vi "CRC.vi"(7 "Byte_order":enum16{"Windows", "DSP"}(ring), 10 "String in":string) -> (1 "CRC16":string, 2 "CRC16":u16 format="%04x", 4 "calculated from #":i32)   [LabVIEW 2017, in "ZBOX_IS.lvlib"]
uses:
  ZBOX_IS.lvlib
panel:
  out "Data in 2":u16[](array[numeric]) format="%02x"
  out "Data in":u8[](array[numeric]) format="%02x"
  out "Data in":u8[](array[numeric]) format="%02x"
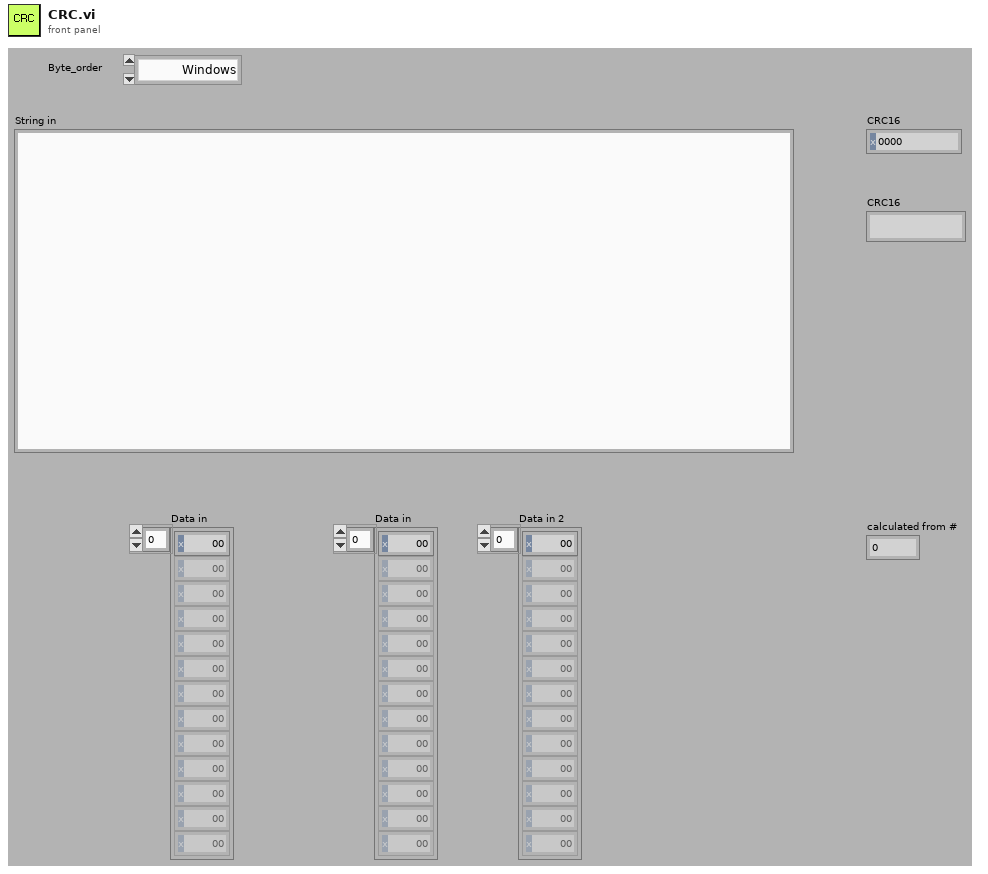
[diagram p1: front panel]
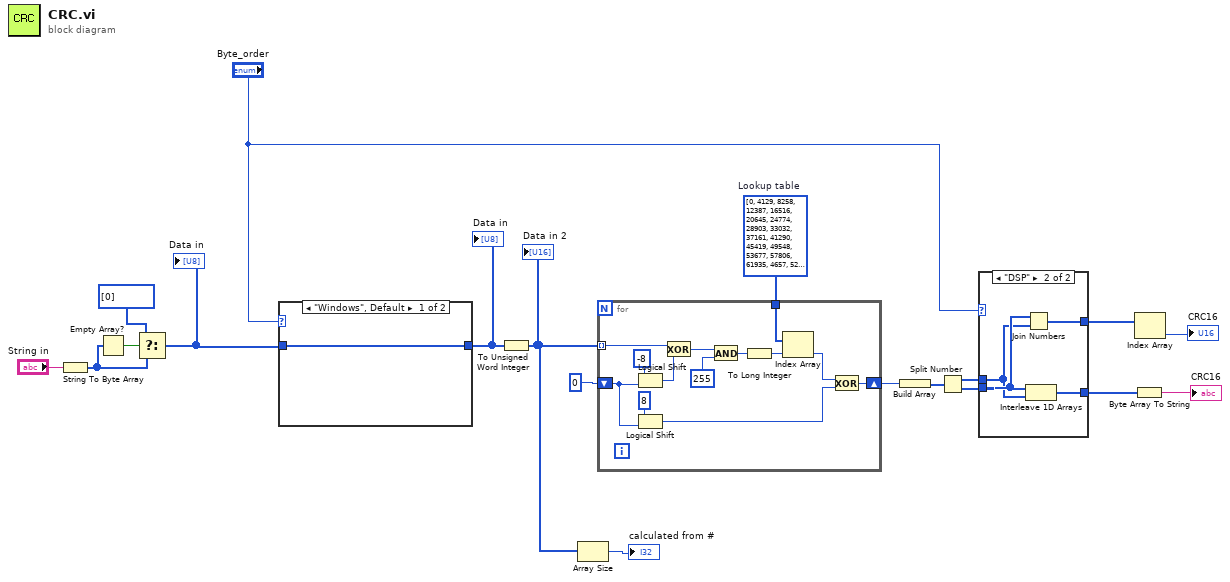
[diagram p0: block diagram]
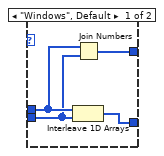
[diagram p2: hidden frame]
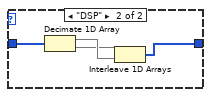
[diagram p3: hidden frame]
diagram:
  w18 = u16[] [0, 4129, 8258, 12387, 16516, 20645, 24774, 28903, 33032, 37161, 41290, 45419, 49548, 53677, 57806, 61935, 4657, 528, 12915, 8786, 21173, 17044, 29431, 25302, 37689, 33560, 45947, 41818, 54205, 50076, 62463, 58334, 9314, 13379, 1056, 5121, 25830, 29895, 17572, 21637, 42346, 46411, 34088, 38153, 58862, 62927, 50604, 54669, 13907, 9842, 5649, 1584, 30423, 26358, 22165, 18100, 46939, 42874, 38681, 34616, 63455, 59390, 55197, 51132, 18628, 22757, 26758, 30887, 2112, 6241, 10242, 14371, 51660, 55789, 59790, 63919, 35144, 39273, 43274, 47403, 23285, 19156, 31415, 27286, 6769, 2640, 14899, 10770, 56317, 52188, 64447, 60318, 39801, 35672, 47931, 43802, 27814, 31879, 19684, 23749, 11298, 15363, 3168, 7233, 60846, 64911, 52716, 56781, 44330, 48395, 36200, 40265, 32407, 28342, 24277, 20212, 15891, 11826, 7761, 3696, 65439, 61374, 57309, 53244, 48923, 44858, 40793, 36728, 37256, 33193, 45514, 41451, 53516, 49453, 61774, 57711, 4224, 161, 12482, 8419, 20484, 16421, 28742, 24679, 33721, 37784, 41979, 46042, 49981, 54044, 58239, 62302, 689, 4752, 8947, 13010, 16949, 21012, 25207, 29270, 46570, 42443, 38312, 34185, 62830, 58703, 54572, 50445, 13538, 9411, 5280, 1153, 29798, 25671, 21540, 17413, 42971, 47098, 34713, 38840, 59231, 63358, 50973, 55100, 9939, 14066, 1681, 5808, 26199, 30326, 17941, 22068, 55628, 51565, 63758, 59695, 39368, 35305, 47498, 43435, 22596, 18533, 30726, 26663, 6336, 2273, 14466, 10403, 52093, 56156, 60223, 64286, 35833, 39896, 43963, 48026, 19061, 23124, 27191, 31254, 2801, 6864, 10931, 14994, 64814, 60687, 56684, 52557, 48554, 44427, 40424, 36297, 31782, 27655, 23652, 19525, 15522, 11395, 7392, 3265, 61215, 65342, 53085, 57212, 44955, 49082, 36825, 40952, 28183, 32310, 20053, 24180, 11923, 16050, 3793, 7920]  # Lookup table
  n1 = String To Byte Array(string="String in") -> (unsigned byte array=w17:u8[])
  n2 = Empty Array?(array=w17) -> (empty?=w15:bool)
  n3 = Select(t=u8[] [0], s=w15, f=w17) -> (s? t:f=w12:u8[])
  "Data in" <- w12
  n4 = case shown="\"Windows\", Default" "Byte_order" {
    tunnel: w12 -> [w20 w22]
    tunnel: [w20 w21] -> w11
    frame "Windows", Default {
    }
    frame "DSP" {
      n5 = Decimate 1D Array(w22) -> (w24:u8[], w23:u8[])
      n6 = Interleave 1D Arrays(w23, w24) -> (w21:u8[])
    }
  }
  "Data in" <- w11
  n7 = To Unsigned Word Integer(number=w11) -> (unsigned 16bit integer=w2:u16[])
  "Data in 2" <- w2
  n8 = Array Size(array=w2) -> (size(s)=→"calculated from #":i32)
  n9 = for {
    tunnel: w2 -> [w37] mode=indexing
    tunnel: w18 -> [w32]
    shift-right: [w28] -> w10
    shift-left: u16 0 ("CRC16 Buffer") -> [w26]
    n10 = Logical Shift(y=-8 ("x"), x=w26) -> (x << y=w36:u16)
    n11 = Logical Shift(y=8, x=w26) -> (x << y=w29:u16)
    n12 = Exclusive Or(1:w36, 2:w37) -> (0:w35:u16)
    n13 = And(x=w35, y=u16 255) -> (x .and. y?=w33:u16)
    n14 = To Long Integer(number=w33) -> (32bit integer=w31:i32)
    n15 = Index Array(array=w32, index=w31) -> (element=w30:u16)
    n16 = Exclusive Or(1:w29, 2:w30) -> (0:w28:u16)
  }
  n17 = Build Array(w10) -> (w7:u16[])
  n18 = Split Number(x=w7) -> (hi(x)=w9:u8[], lo(x)=w8:u8[])
  n19 = case shown="\"DSP\"" "Byte_order" {
    tunnel: w9 -> [w40 w43]
    tunnel: w8 -> [w39 w44]
    tunnel: [w41 w45] -> w6
    tunnel: [w38 w42] -> w4
    frame "Windows", Default {
      n20 = Interleave 1D Arrays(w40, w39) -> (w41:u8[])
      n21 = Join Numbers(hi=w40, lo=w39) -> ((hi.lo)=w38:u16[])
    }
    frame "DSP" {
      n22 = Join Numbers(hi=w44, lo=w43) -> ((hi.lo)=w42:u16[])
      n23 = Interleave 1D Arrays(w44, w43) -> (w45:u8[])
    }
  }
  n24 = Byte Array To String(unsigned byte array=w6) -> (string=→"CRC16":string)
  n25 = Index Array(array=w4) -> (element=→"CRC16":u16)  [unwired: 1 in]
